vi "Example Graph - ObjectTemperature Callback.vi"(4 "ObjectTemperature":refnum<user-event>, 5 "Event Data":cluster{"sender":refnum<k24>, "temperature":i16}, 6 "Control Ref":refnum<k24>, 7 "Event Common Data":T1) -> ()   [LabVIEW 2010]
uses:
  C:/tf/play/labview/Tinkerforge.dll
  Tinkerforge.dll
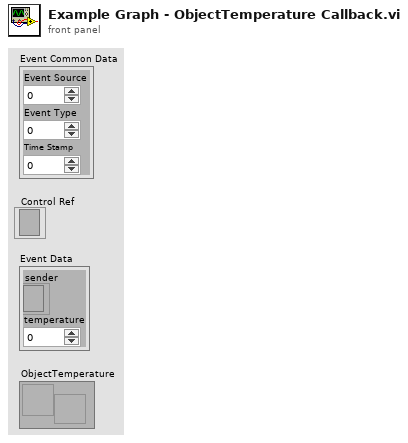
[diagram p1: front panel]
types:
  T1 = cluster{"Event Source":i32, "Event Type":u32, "Time Stamp":u32}
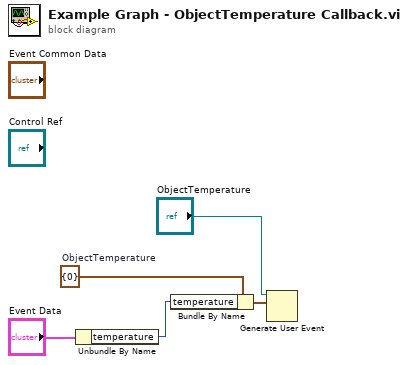
[diagram p0: block diagram]
diagram:
  w4 = cluster{"temperature":i16} {"temperature"=0}  # ObjectTemperature
  n1 = Unbundle By Name("Event Data") -> ("temperature"=w3:i16)
  n2 = Bundle By Name(cluster=w4, "temperature"=w3) -> (w2:cluster{"temperature":i16})
  n3 = Generate User Event(user event="ObjectTemperature", event data cluster=w2) -> ()  [unwired: 1 in, 2 out]
